vi "AutoLin Protokoll.vi"(10 "Sollwerte":sgl[](array[numeric]), 11 "Lin-Eing.":sgl[][](array[numeric])) -> (0 "XY-Graph (roh/lin)":cluster{"eine Kurve":sgl[], dbl[]}[](array[cluster]), 2 "Messdaten und Fehler":string[][](array[string]), 3 "Ergebnis":string[][](array[string]))   [LabVIEW 2015]
doc: "Bereitet die Messdaten und die Linearisierungs-Polynom-Daten zu zwei 2D-Arrays (String) auf,die direkt in einem Tabellenelement angezeigt oder in einer Textdatei gespeichert werden können."
uses:
  Linearisierung/AutoLin Protokoll/AutoLin Protokoll.lvlib
  Linearisierung/Linearisierung.lvlib
  Linearisierung/Aktionen Polynom Daten speichern.ctl
  Messdaten/Aktionen FGV Messdaten.ctl
  Messdaten/Messdaten.lvlib
  <vilib>/Analysis/NI_AALPro.lvlib
  Linearisierung/AutoLin Protokoll-Info.ctl
  Eingabetabelle.ctl
  Neue Linearisierung.lvlib
panel:
  in  "Eingabetabelle":T1
  in  "Protokoll-Info":T2
  in  "Polynom-Ordnung":i32
  in  "F_max in %":sgl
  # "Gasteiler (ppm)"
  # "Messgerät (ppm)"
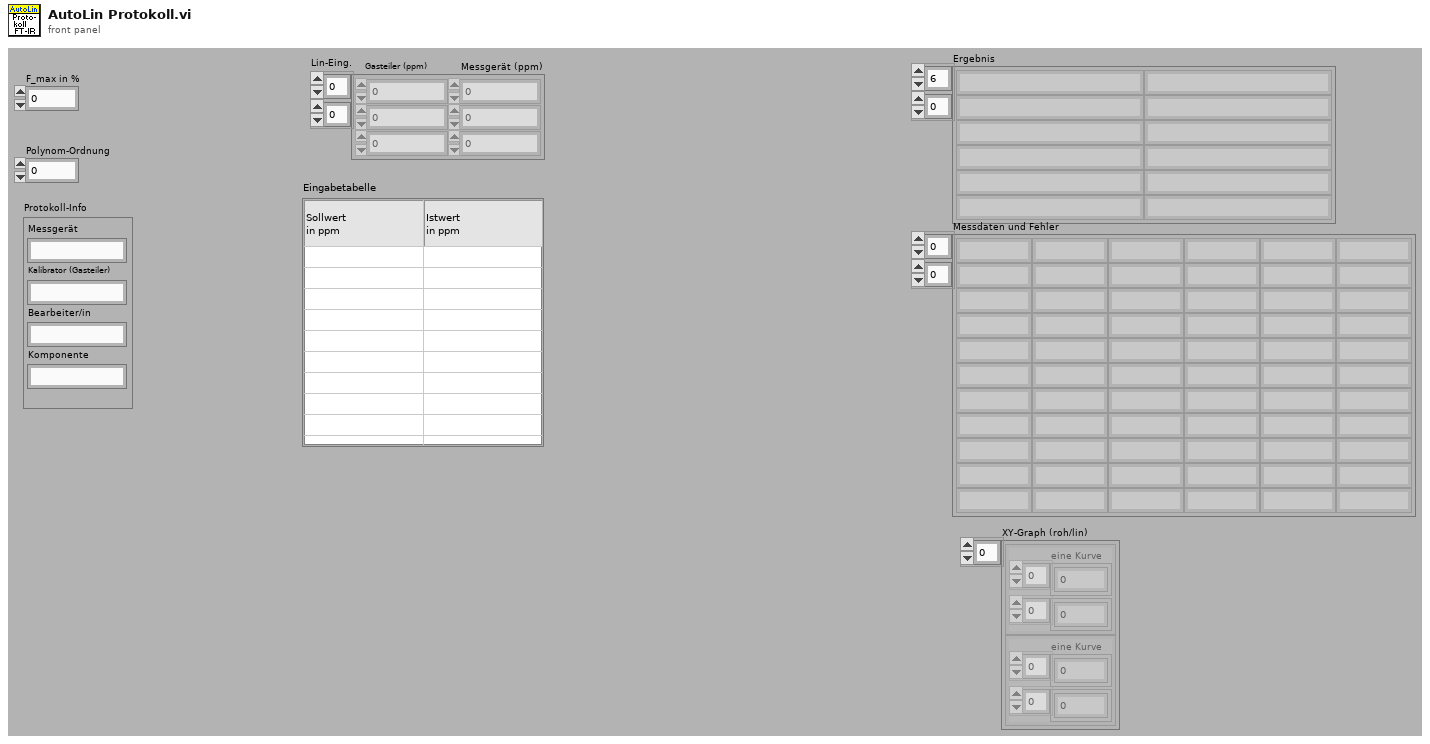
[diagram p1: front panel]
types:
  T1 = typedef "Neue Linearisierung.lvlib/Eingabetabelle.ctl" = string[][]
  T2 = typedef "Linearisierung.lvlib/AutoLin Protokoll-Info.ctl" = cluster{"Messgerät":string, "Kalibrator (Gasteiler)":string, "Bearbeiter/in":string, "Komponente":string}
  T3 = typedef "Messdaten.lvlib/Aktionen FGV Messdaten.ctl" = enum16{"lesen", "schreiben", "löschen", "Mittelwerte", "Komponente"}
  T4 = typedef "Linearisierung.lvlib/Aktionen Polynom Daten speichern.ctl" = enum16{"lesen", "laden", "speichern", "schreiben1", "schreiben alle", "Liste erstellen"}
  T5 = typedef "Linearisierung.lvlib/AutoLin Lin-Polynom.ctl" = cluster{"Messgerät":string, "Kalibrator (Gasteiler)":string, "Bearbeiter/in":string, "Komponente":string, "Zeitstempel":timestamp, "F_max gefordert (%)":sgl, "F_max in %":sgl, "F_max in ppm":sgl, "Vorschlag Ordnung":i32, "Polynom OK":bool, "Polynomkoeff.":sgl[], "Prüfgas Konzentration":sgl, "Pfad1":string, "Pfad_LIN":string}
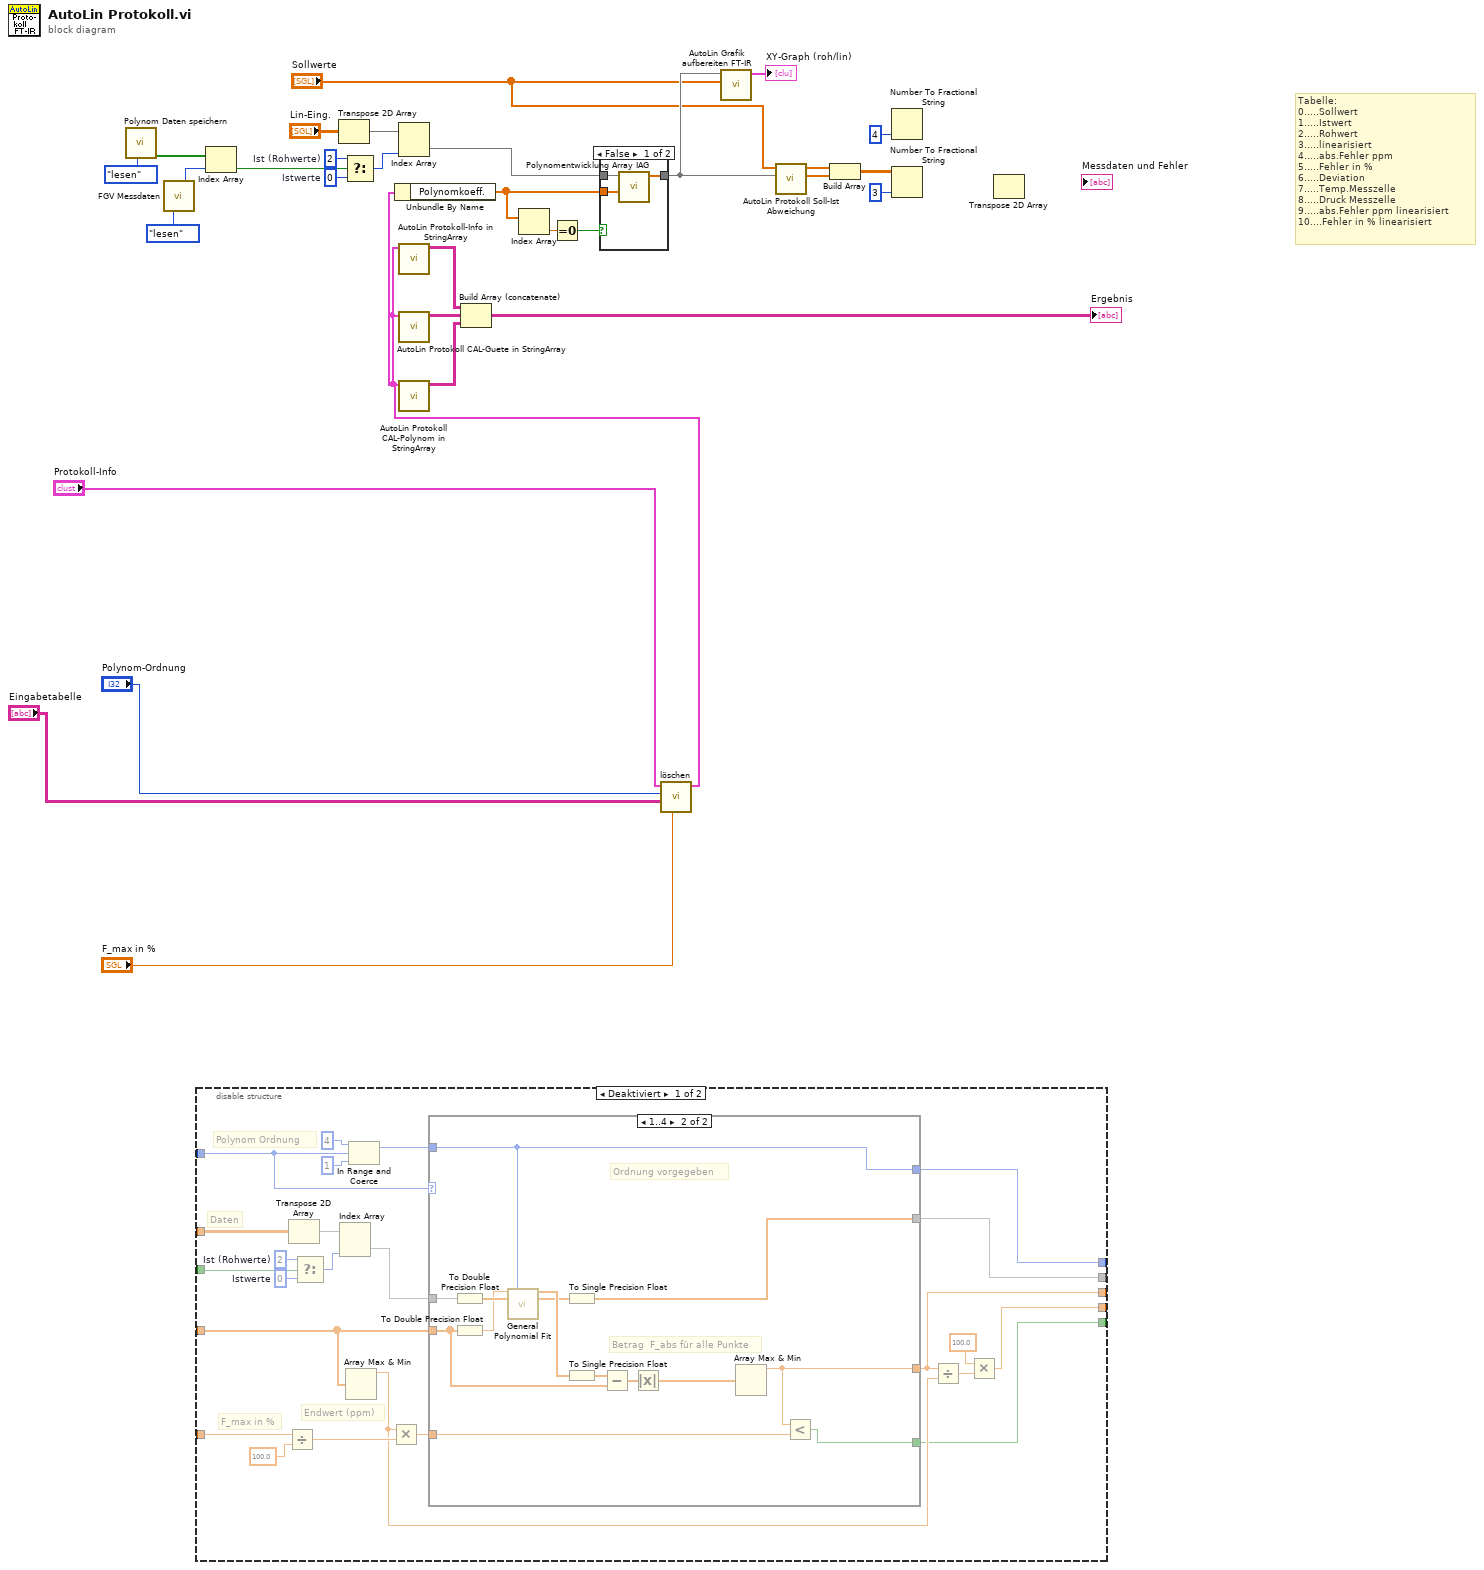
[diagram p0: block diagram]
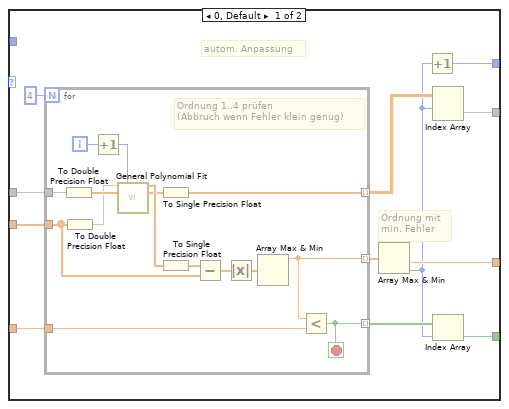
[diagram p2: hidden frame]
diagram:
  w10 = 0  # Istwerte
  w9 = 2  # Ist (Rohwerte)
  # "Tabelle:\n0.....Sollwert\n1.....Istwert\n2.....Rohwert\n3.....linearisiert\n4.....abs.Fehler ppm\n5.....Fehler in %\n6.....Deviation\n7.....Temp.Messzelle\n8.....Druck Messzelle\n9.....abs.Fehler ppm linearisiert\n10....Fehler in % linearisiert"
  n1 = call "Polynom Daten speichern.vi"("Aktionen"=Aktionen_Polynom_Daten_speichern."lesen") -> ("Aktiv"=w13:bool[])  [unwired: 7 in, 3 out]
  n2 = call "FGV Messdaten.vi"("Aktionen"=Aktionen_FGV_Messdaten."lesen") -> ("Komponente"=w11:u16)  [unwired: 6 in, 8 out]
  n3 = disable-structure shown="Deaktiviert" {
    disable-tunnel: _ -> [w53 _]
    disable-tunnel: [w45 _] -> _
    disable-tunnel: [w44 _] -> _
    disable-tunnel: [w43 _] -> _
    disable-tunnel: [w42 _] -> _
    disable-tunnel: _ -> [w41 _]
    disable-tunnel: [w40 _] -> _
    disable-tunnel: _ -> [w39 _]
    disable-tunnel: _ -> [w38 _]
    disable-tunnel: _ -> [w33 _]
    frame Disabled {
      w36 = 0  # Istwerte
      w34 = 2  # Ist (Rohwerte)
      # "Polynom Ordnung"
      # "Daten"
      # "F_max in %"
      # "Endwert (ppm)"
      n4 = Divide(x=w41, y=sgl 100.0) -> (x/y=w51:sgl)
      n5 = Transpose 2D Array(2D array=w38) -> (transposed array=w37:dbl[][])
      n6 = Select(t=w34, s=w33, f=w36) -> (s? t:f=w35:i32)
      n7 = Index Array(array=w37, index (col)=w35) -> (element=w46:dbl[])  [unwired: 1 in]
      n8 = Array Max & Min(array=w39) -> (max value=w49:dbl)  [unwired: 3 out]
      n9 = In Range and Coerce(upper limit=4 ("Obergrenze"), x=w53, lower limit=1 ("Untergrenze")) -> (coerced(x)=w54:i32)  [unwired: 1 out]
      n10 = Multiply(x=w49, y=w51) -> (x*y=w50:dbl)
      n11 = case shown="1..4" w53 {
        tunnel: w46 -> [w68 w91]
        tunnel: w39 -> [w67 w89]
        tunnel: w54 -> [_ w92]
        tunnel: w50 -> [w65 w97]
        tunnel: [w62 w84] -> w40
        tunnel: [w64 w94] -> w44
        tunnel: [w59 w93] -> w42
        tunnel: [w61 w92] -> w45
        frame 0, Default {
          # "Ordnung mit\nmin. Fehler"
          # "autom. Anpassung"
          n12 = for {
            N: 4 -> [_]
            tunnel: w68 -> [w76]
            tunnel: w67 -> [w74]
            tunnel: [w70] -> w63 mode=indexing
            tunnel: w65 -> [w81]
            tunnel: [w77] -> w57 mode=indexing
            tunnel: [w78] -> w60 mode=indexing
            i -> [w83]
            stop <- w78 stop-if-true
            # "Ordnung 1..4 prüfen\n(Abbruch wenn Fehler klein genug)"
            n13 = To Double Precision Float(number=w76) -> (double precision float=w75:dbl[])
            n14 = To Double Precision Float(number=w74) -> (double precision float=w73:dbl)
            n15 = Increment(x=w83) -> (x+1=w79:i32)
            n16 = call <vilib>:"General Polynomial Fit.vi"("Y"=w73, "polynomial order"=w79, "X"=w75) -> ("Best Polynomial Fit"=w72:dbl[], "Polynomial Coefficients"=w69:dbl[])  [unwired: 9 in, 2 out]
            n17 = To Single Precision Float(number=w69) -> (single precision float=w70:sgl[])
            n18 = To Single Precision Float(number=w72) -> (single precision float=w71:sgl[])
            n19 = Subtract(x=w71, y=w74) -> (x-y=w82:sgl[])
            n20 = Absolute Value(x=w82) -> (abs(x)=w80:sgl[])
            n21 = Array Max & Min(array=w80) -> (max value=w77:sgl)  [unwired: 3 out]
            n22 = Less?(x=w77, y=w81) -> (x < y?=w78:bool)
          }
          n23 = Array Max & Min(array=w57) -> (min value=w64:sgl, min index (indices)=w58:i32)  [unwired: 2 out]
          n24 = Increment(x=w58) -> (x+1=w61:i32)
          n25 = Index Array(array=w63, index (row)=w58) -> (element=w62:sgl[])  [unwired: 1 in]
          n26 = Index Array(array=w60, index=w58) -> (element=w59:bool)
        }
        frame 1..4 {
          # "Betrag  F_abs für alle Punkte"
          # "Ordnung vorgegeben"
          n27 = To Double Precision Float(number=w91) -> (double precision float=w90:dbl[])
          n28 = To Double Precision Float(number=w89) -> (double precision float=w88:dbl)
          n29 = call <vilib>:"General Polynomial Fit.vi"("Y"=w88, "polynomial order"=w92, "X"=w90) -> ("Best Polynomial Fit"=w87:dbl[], "Polynomial Coefficients"=w85:dbl[])  [unwired: 9 in, 2 out]
          n30 = To Single Precision Float(number=w85) -> (single precision float=w84:sgl[])
          n31 = To Single Precision Float(number=w87) -> (single precision float=w86:sgl[])
          n32 = Subtract(x=w86, y=w89) -> (x-y=w96:sgl[])
          n33 = Absolute Value(x=w96) -> (abs(x)=w95:sgl[])
          n34 = Array Max & Min(array=w95) -> (max value=w94:sgl)  [unwired: 3 out]
          n35 = Less?(x=w94, y=w97) -> (x < y?=w93:bool)
        }
      }
      n36 = Divide(x=w44, y=w49) -> (x/y=w48:dbl)
      n37 = Multiply(x=sgl 100.0, y=w48) -> (x*y=w43:dbl)
    }
    frame Enabled {
    }
  }
  n38 = Index Array(array=w13, index=w11) -> (element=w8:bool)
  n39 = Transpose 2D Array(2D array="Lin-Eing.") -> (transposed array=w18:sgl[][])
  n40 = Select(t=w9, s=w8, f=w10) -> (s? t:f=w7:i32)
  n41 = Index Array(array=w18, index (col)=w7) -> (element=w28:sgl[])  [unwired: 1 in]
  n42 = call "löschen.vi"("F_max in %"="F_max in %", "Eingabetabelle"="Eingabetabelle", "Polynom-Ordnung"="Polynom-Ordnung", "Protokoll-Info"="Protokoll-Info") -> ("Polynomanpassung"=w1:T5)  [unwired: 7 in]
  n43 = Unbundle By Name(w1) -> ("Polynomkoeff."=w20:sgl[])
  n44 = call "AutoLin Protokoll-Info in StringArray.vi"("Lin-Polynom"=w1) -> ("Protokoll-Info-String"=w29:string[][])  [unwired: 10 in]
  n45 = call "AutoLin Protokoll CAL-Guete in StringArray.vi"("Lin-Polynom"=w1) -> ("Lin-Güte (Protokoll)"=w32:string[][])  [unwired: 10 in]
  n46 = call "AutoLin Protokoll CAL-Polynom in StringArray.vi"("Lin-Polynom"=w1) -> ("LinPolynom (Protokoll)"=w31:string[][])  [unwired: 10 in]
  n47 = Build Array (concatenate)(w29, w32, w31) -> (→"Ergebnis":string[][])
  n48 = Index Array(array=w20) -> (element=w22:sgl)  [unwired: 1 in]
  n49 = Equal To 0?(x=w22) -> (x = 0?=w21:bool)
  n50 = case shown="False" w21 {
    tunnel: w20 -> [w100 _]
    tunnel: w28 -> [w99 w101]
    tunnel: [w98 w101] -> w17
    frame False {
      n51 = call "Polynomentwicklung Array IAG.vi"("P(x) 2"=w100, "A"=w99) -> ("P(A)"=w98:sgl[])  [unwired: 9 in]
    }
    frame True {
    }
  }
  n52 = call "AutoLin Grafik aufbereiten FT-IR.vi"("Sollwerte"="Sollwerte", "Istwerte"=w17) -> ("XY-Graph (roh/lin)"=→"XY-Graph (roh/lin)":cluster{"eine Kurve":sgl[], dbl[]}[])  [unwired: 9 in]
  n53 = call "AutoLin Protokoll Soll-Ist Abweichung.vi"("Istwerte (ppm)"=w17, "Sollwerte (ppm)"="Sollwerte") -> ("% vom Sollwert"=w26:sgl[], "abs. Fehler (ppm)"=w6:sgl[])  [unwired: 7 in, 1 out]
  n54 = Build Array(w6, w26) -> (w25:sgl[][])
  n55 = Number To Fractional String(precision (6)=i16 4 ("Genauigkeit (6)")) -> (number=w27:dbl)  [unwired: 2 in, 1 out]
  n56 = Number To Fractional String(number=w25, precision (6)=i16 3 ("Genauigkeit (6)")) -> ()  [unwired: 2 in, 1 out]
  n57 = Transpose 2D Array() -> ()  [unwired: 1 in, 1 out]
